vi "AI Voltage Single Channel Measurement.vi"(6 "Measurement Mode":T2(ring)=enum."Single Channel : Multiple Samples", 8 "error in (no error)":errorcluster, 9 "Timing Settings":T1={"Sample Rate"=1000.0, "Number of Samples"=100}, 10 "Channel Settings":T3={"Min Value"=-5.0, "Max Value"=5.0, "Terminal Configuration"=-1} {"Terminal Configuration" items=["default"=-1, "RSE"=10083, "NRSE"=10078, "Differential"=10106, "Pseudodifferential"=12529]}, 11 "Physical Channel":tag="Dev1/ai0") -> (0 "error out":errorcluster, 1 "Actual Sample Rate":dbl=1000.0 format="%0.2f", 2 "Waveform Graph":waveform(dbl)(graph))   [LabVIEW 2022 SP3, in "niMIO.lvclass"]
uses:
  niMIO.lvclass
  Type Definitions/AI Channel Settings.ctl
  Type Definitions/Timing Settings.ctl
  <vilib>/DAQmx/read.llb/DAQmx Read (Analog Wfm 1Chan NSamp).vi
  <vilib>/DAQmx/read.llb/DAQmx Read (Analog Wfm 1Chan 1Samp).vi
  <vilib>/DAQmx/create/channels.llb/DAQmx Create Channel (AI-Voltage-Basic).vi
  <vilib>/DAQmx/configure/timing.llb/DAQmx Timing (Sample Clock).vi
  <vilib>/DAQmx/miscellaneous.llb/DAQmx Fill In Error Info.vi
  <resource>/objmgr/daqmx.rc
panel:
  out "niMIO out":refnum<class "niMIO.lvclass">
  in  "niMIO in":refnum<class "niMIO.lvclass">
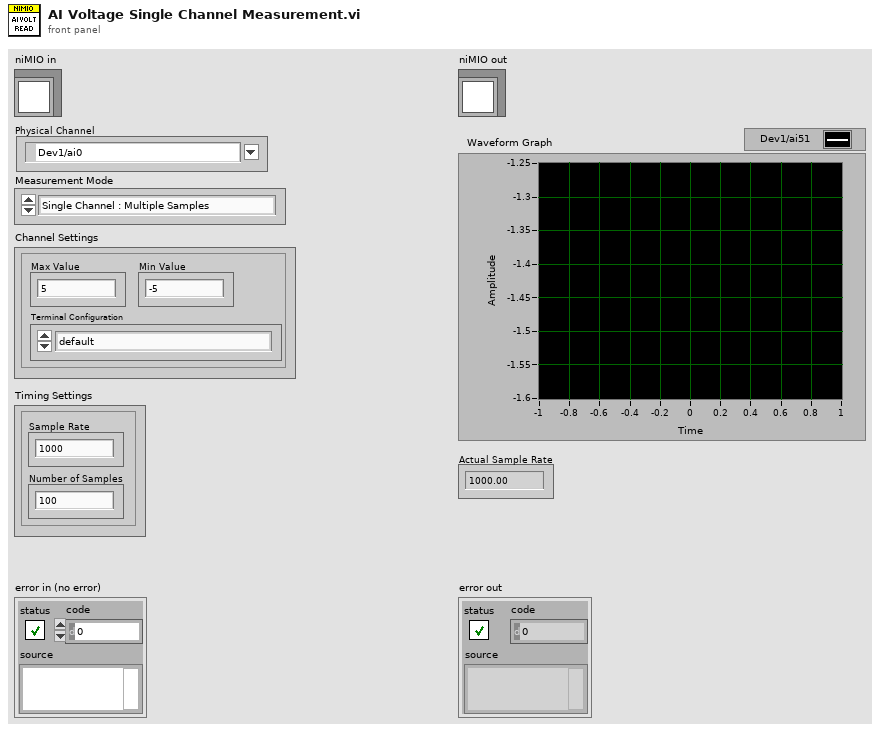
[diagram p1: front panel]
types:
  T1 = typedef "niMIO.lvclass/Timing Settings.ctl" = cluster{"Sample Rate":dbl, "Number of Samples":i32}
  T2 = enum16{"Single Channel : Single Sample", "Single Channel : Multiple Samples"}
  T3 = typedef "niMIO.lvclass/AI Channel Settings.ctl" = cluster{"Min Value":dbl, "Max Value":dbl, "Terminal Configuration":i32}
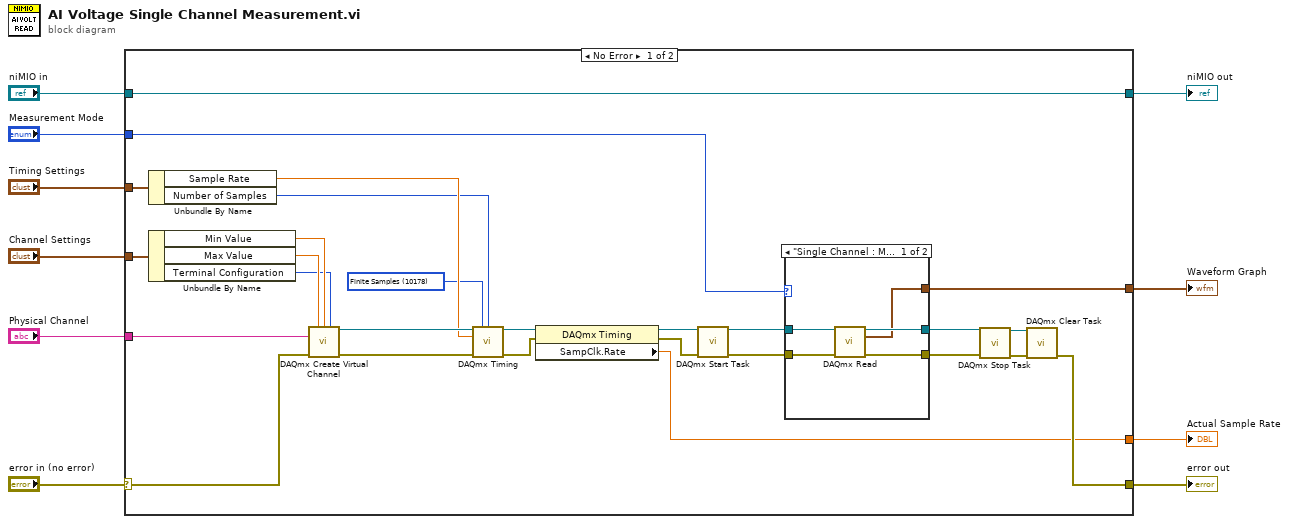
[diagram p0: block diagram]
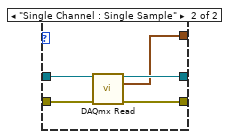
[diagram p2: hidden frame]
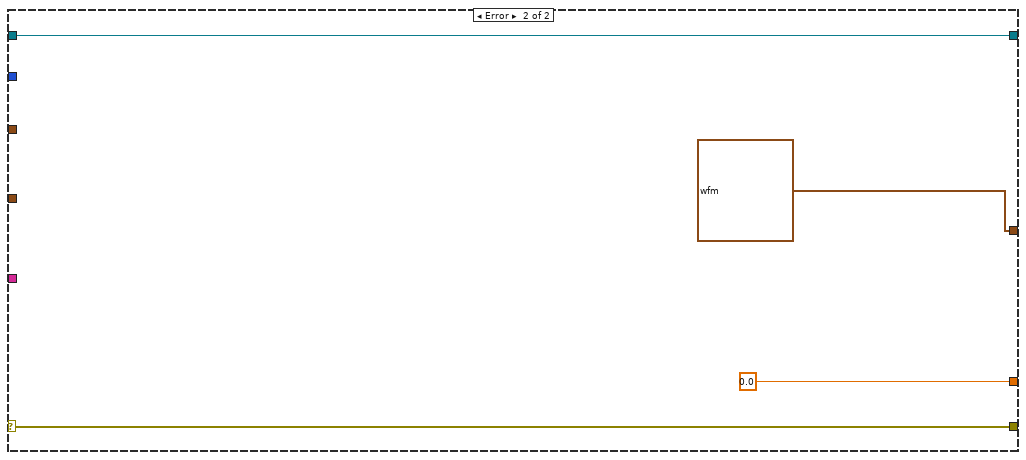
[diagram p3: hidden frame]
diagram:
  n1 = case shown="No Error" "error in (no error)" {
    selector: "error in (no error)" -> [w25 w51]
    tunnel: [w35 w51] -> w9
    tunnel: [w37 w50] -> w1
    tunnel: "niMIO in" -> [w37 w50]
    tunnel: "Channel Settings" -> [w28 _]
    tunnel: "Timing Settings" -> [w24 _]
    tunnel: [w17 0.0 ("SampClk.Rate")] -> w8
    tunnel: "Measurement Mode" -> [w16 _]
    tunnel: [w15 waveform(dbl) {"t0"=timestamp(0 s since 1904-01-01), "dt"=1.0, "Y"=[]} ("data")] -> w5
    tunnel: "Physical Channel" -> [w13 _]
    frame No Error {
      w22 = 10178 items=["Finite Samples"=10178, "Continuous Samples"=10123, "Hardware Timed Single Point"=12522] ("sample mode")
      n2 = Unbundle By Name(w24) -> ("Sample Rate"=w23:dbl, "Number of Samples"=w14:i32)
      n3 = Unbundle By Name(w28) -> ("Min Value"=w27:dbl, "Max Value"=w26:dbl, "Terminal Configuration"=w12:i32)
      n4 = call-poly <vilib>:"DAQmx Create Virtual Channel.vi"("maximum value"=w26, "minimum value"=w27, "input terminal configuration"=w12, "physical channels"=w13, "error in"=w25) -> ("task out"=w30:refnum<k21>, "error out"=w34:errorcluster)  [unwired: 9 in]
      n5 = call-poly <vilib>:"DAQmx Timing.vi"("task/channels in"=w30, "sample mode"=w22, "samples per channel"=w14, "rate"=w23, "error in"=w34) -> ("task out"=w19:refnum<k21>, "error out"=w20:errorcluster)  [unwired: 9 in]
      n6 = property class="DAQmx Timing"(reference=w19, error in=w20) -> (reference out=w18:refnum<k21>, error out=w21:errorcluster, "SampClk.Rate"=w17:dbl)
      n7 = call <vilib>:"DAQmx Start Task.vi"("task/channels in"=w18, "error in"=w21) -> ("task out"=w29:refnum<k21>, "error out"=w11:errorcluster)  [unwired: 12 in]
      n8 = case shown="\"Single Channel : Multiple Samples\"" w16 {
        tunnel: w11 -> [w42 w47]
        tunnel: [w41 w46] -> w33
        tunnel: [w40 w45] -> w32
        tunnel: w29 -> [w39 w44]
        tunnel: [w38 w43] -> w15
        frame "Single Channel : Multiple Samples" {
          n9 = call-poly <vilib>:"DAQmx Read.vi"("task/channels in"=w39, "error in"=w42) -> ("task out"=w40:refnum<k21>, "data"=w38:waveform(dbl), "error out"=w41:errorcluster)  [unwired: 11 in]
        }
        frame "Single Channel : Single Sample" {
          n10 = call-poly <vilib>:"DAQmx Read.vi"("task/channels in"=w44, "error in"=w47) -> ("task out"=w45:refnum<k21>, "data"=w43:waveform(dbl), "error out"=w46:errorcluster)  [unwired: 11 in]
        }
      }
      n11 = call <vilib>:"DAQmx Stop Task.vi"("task/channels in"=w32, "error in"=w33) -> ("task out"=w31:refnum<k21>, "error out"=w36:errorcluster)  [unwired: 12 in]
      n12 = call <vilib>:"DAQmx Clear Task.vi"("task in"=w31, "error in"=w36) -> ("error out"=w35:errorcluster)  [unwired: 13 in]
    }
    frame Error {
    }
  }
  "error out" <- w9
  "Actual Sample Rate" <- w8
  "Waveform Graph" <- w5
  "niMIO out" <- w1
